vi "SLT Filter Process Information.vi"(0 "All Process Handles":i32[](array[numeric]), 1 "Process Names to Monitor":string[](array[string]), 2 "Process IDs to Monitor":u32[](array[numeric]), 5 "All Process IDs":u32[](array[numeric]), 7 "All Process Names":string[](array[string]), 11 "error in (no error)":errorcluster) -> (4 "Filtered Process Handles":i32[](array[numeric]), 6 "Filtered Process IDs":u32[](array[numeric]), 8 "Filtered Process Names":string[](array[string]), 10 "Number of Processes":i32, 15 "error out":errorcluster)   [LabVIEW 2013, in "ProcessInfo.lvlib"]
uses:
  ProcessInfo.lvlib
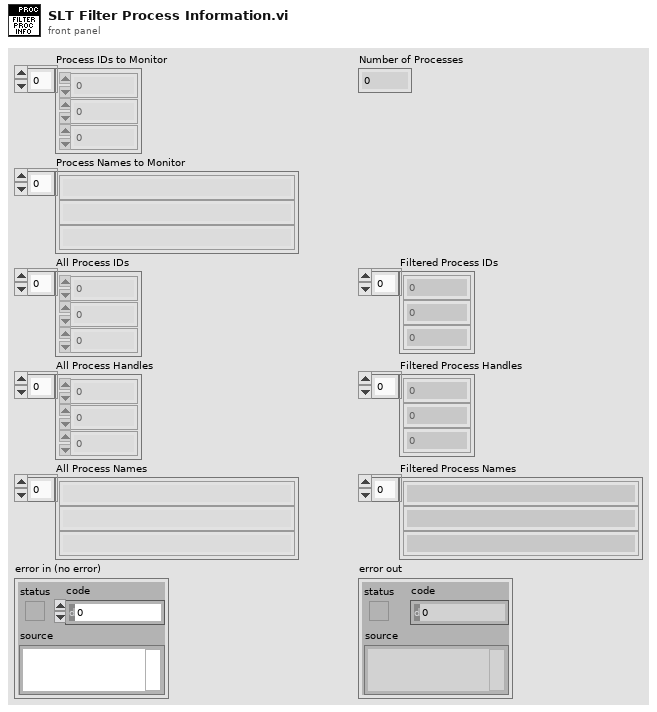
[diagram p1: front panel]
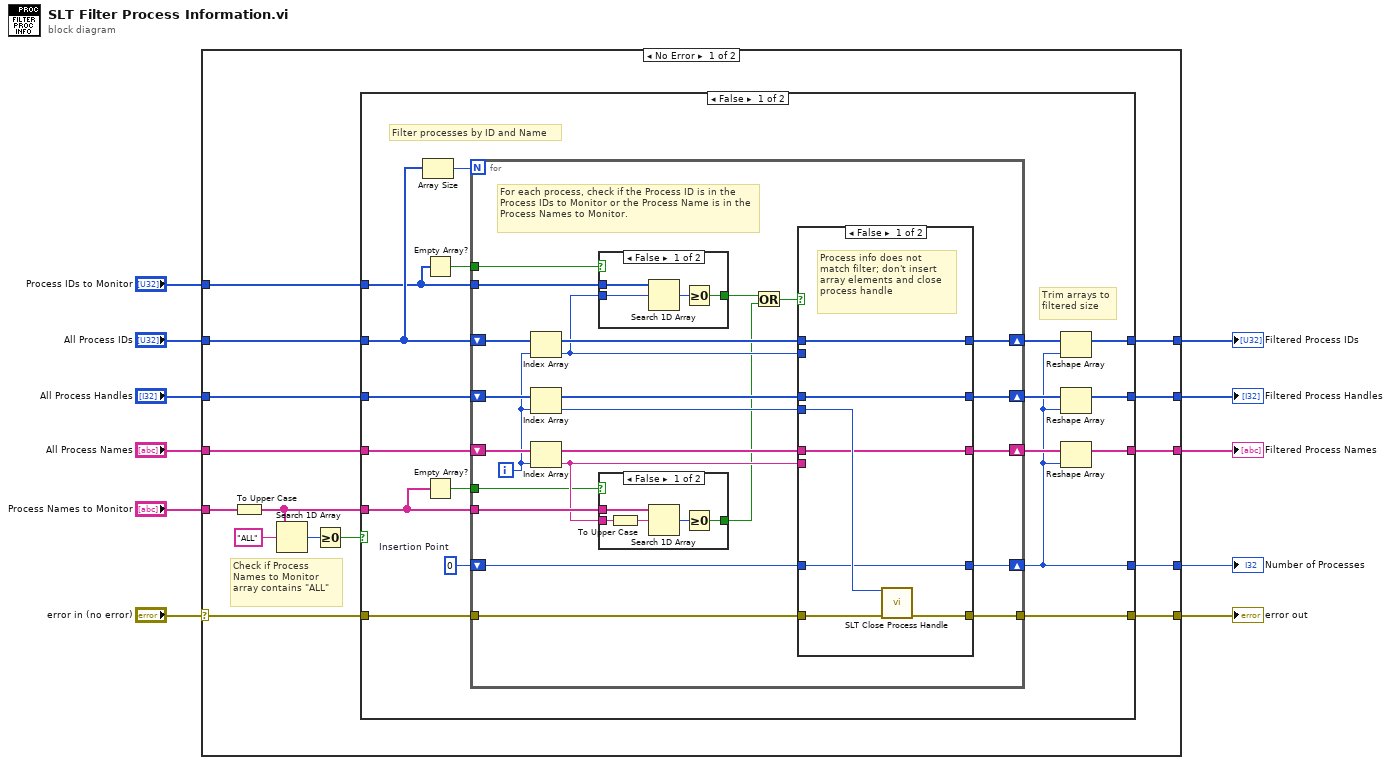
[diagram p0: block diagram]
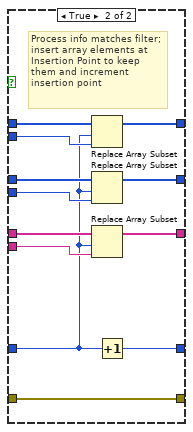
[diagram p4: hidden frame]
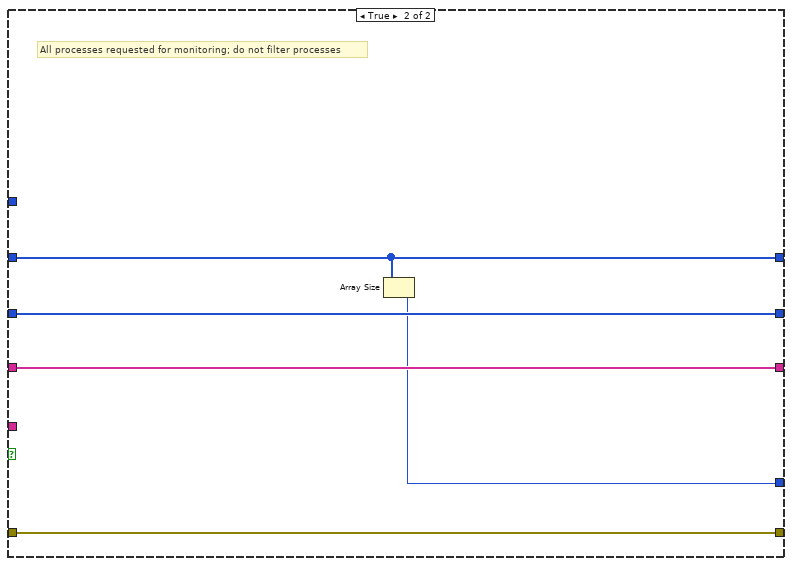
[diagram p5: hidden frame]
diagram:
  n1 = case shown="No Error" "error in (no error)" {
    selector: "error in (no error)" -> [w24 w99]
    tunnel: "Process IDs to Monitor" -> [w18 _]
    tunnel: "All Process Handles" -> [w26 _]
    tunnel: "All Process IDs" -> [w23 _]
    tunnel: "All Process Names" -> [w25 _]
    tunnel: [w22 w99] -> w5
    tunnel: "Process Names to Monitor" -> [w15 _]
    tunnel: [w21 _] -> w8
    tunnel: [w20 _] -> w9
    tunnel: [w19 _] -> w10
    tunnel: [w12 _] -> w11
    frame No Error {
      # "Check if Process Names to Monitor array contains \"ALL\""
      n2 = To Upper Case(1:w15) -> (0:w14:string[])
      n3 = Search 1D Array(1D array=w14, element="ALL") -> (index of element=w17:i32)  [unwired: 1 in]
      n4 = Greater Or Equal To 0?(x=w17) -> (x >= 0?=w13:bool)
      n5 = case shown="False" w13 {
        tunnel: w26 -> [w44 w98]
        tunnel: w25 -> [w43 w97]
        tunnel: w24 -> [w41 w96]
        tunnel: w23 -> [w39 w95]
        tunnel: [w38 w96] -> w22
        tunnel: [w34 w95] -> w21
        tunnel: [w33 w98] -> w20
        tunnel: [w32 w97] -> w19
        tunnel: w18 -> [w31 _]
        tunnel: w14 -> [w28 _]
        tunnel: [w27 w94] -> w12
        frame False {
          w42 = 0  # Insertion Point
          # "Trim arrays to filtered size"
          # "Filter processes by ID and Name"
          n6 = Array Size(array=w39) -> (size(s)=w40:i32)
          n7 = Empty Array?(array=w31) -> (empty?=w30:bool)
          n8 = Empty Array?(array=w28) -> (empty?=w29:bool)
          n9 = for {
            N: w40 -> [_]
            tunnel: w31 -> [w65]
            shift-right: [w48] -> w27
            shift-left: w42 -> [w53]
            tunnel: w28 -> [w59]
            tunnel: w41 -> [w52]
            shift-right: [w51] -> w37
            shift-left: w39 -> [w64]
            shift-right: [w50] -> w36
            shift-left: w44 -> [w61]
            shift-right: [w49] -> w35
            shift-left: w43 -> [w62]
            tunnel: [w47] -> w38
            tunnel: w30 -> [w46]
            tunnel: w29 -> [w45]
            i -> [w60]
            # "For each process, check if the Process ID is in the Process IDs to Monitor or the Process Name is in the Process Names to Monitor."
            n10 = Index Array(array=w64, index=w60) -> (element=w63:u32)
            n11 = Index Array(array=w61, index=w60) -> (element=w57:i32)
            n12 = Index Array(array=w62, index=w60) -> (element=w58:string)
            n13 = case shown="False" w46 {
              tunnel: w65 -> [w73 _]
              tunnel: w63 -> [w72 _]
              tunnel: [w71 _] -> w55
              frame False {
                n14 = Search 1D Array(1D array=w73, element=w72) -> (index of element=w74:i32)  [unwired: 1 in]
                n15 = Greater Or Equal To 0?(x=w74) -> (x >= 0?=w71:bool)
              }
              frame True {
              }
            }
            n16 = case shown="False" w45 {
              tunnel: w59 -> [w70 _]
              tunnel: w58 -> [w69 _]
              tunnel: [w67 _] -> w54
              frame False {
                n17 = To Upper Case(1:w69) -> (0:w66:string)
                n18 = Search 1D Array(1D array=w70, element=w66) -> (index of element=w68:i32)  [unwired: 1 in]
                n19 = Greater Or Equal To 0?(x=w68) -> (x >= 0?=w67:bool)
              }
              frame True {
              }
            }
            n20 = Or(x=w55, y=w54) -> (x .or. y?=w56:bool)
            n21 = case shown="False" w56 {
              tunnel: w64 -> [w75 w93]
              tunnel: w61 -> [w76 w91]
              tunnel: w62 -> [w77 w89]
              tunnel: w63 -> [_ w92]
              tunnel: w58 -> [_ w88]
              tunnel: w57 -> [w79 w90]
              tunnel: w53 -> [w78 w84]
              tunnel: w52 -> [w80 w82]
              tunnel: [w75 w87] -> w51
              tunnel: [w76 w86] -> w50
              tunnel: [w77 w85] -> w49
              tunnel: [w78 w83] -> w48
              tunnel: [w81 w82] -> w47
              frame False {
                # "Process info does not match filter; don't insert array elements and close process handle"
                n22 = call "SLT Close Process Handle.vi"("handle"=w79, "error in (no error)"=w80) -> ("error out"=w81:errorcluster)  [unwired: 13 in]
              }
              frame True {
                # "Process info matches filter; insert array elements at Insertion Point to keep them and increment insertion point"
                n23 = Replace Array Subset(array=w93, new element=w92, index=w84) -> (w87:u32[])
                n24 = Replace Array Subset(array=w91, new element=w90, index=w84) -> (w86:i32[])
                n25 = Replace Array Subset(array=w89, new element=w88, index=w84) -> (w85:string[])
                n26 = Increment(x=w84) -> (x+1=w83:i32)
              }
            }
          }
          n27 = Reshape Array(w37, w27) -> (w34:u32[])
          n28 = Reshape Array(w36, w27) -> (w33:i32[])
          n29 = Reshape Array(w35, w27) -> (w32:string[])
        }
        frame True {
          # "All processes requested for monitoring; do not filter processes"
          n30 = Array Size(array=w95) -> (size(s)=w94:i32)
        }
      }
    }
    frame Error {
    }
  }
  "error out" <- w5
  "Filtered Process IDs" <- w8
  "Filtered Process Handles" <- w9
  "Filtered Process Names" <- w10
  "Number of Processes" <- w11
